vi "AMI_String_Field Z.vi"(8 "error in (no error)":errorcluster, 11 "String":string="Set Z Axis Magnetic Field 0.100Tesla at 0.030Tesla/min, PAUSE, Wait") -> (0 "error out":errorcluster, 2 "Z Rate":dbl, 3 "Z Field":dbl, 4 "Z H.Wait Stability":bool, 5 "Z Modo Rampa":u16(ring)=1 items=["RAMP", "PAUSE", "PAUSE", "MANUAL DOWN", "ZERO"])   [LabVIEW 2017]
panel:
  out "subString":string
  # "Set Z Axis Magnetic Field 0.100Tesla at 0.030Tesla/min, PAUSE, Wait"
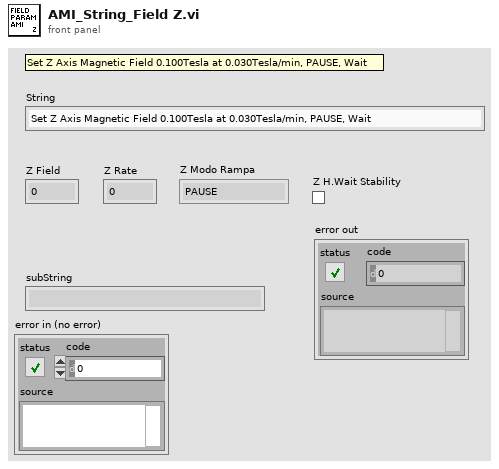
[diagram p1: front panel]
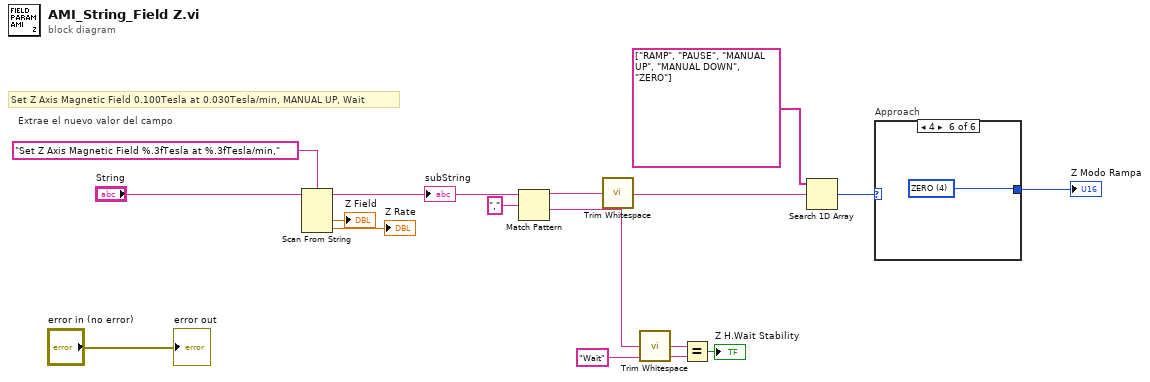
[diagram p0: block diagram]
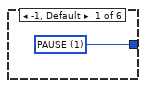
[diagram p2: hidden frame]
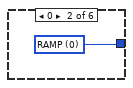
[diagram p3: hidden frame]
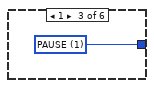
[diagram p4: hidden frame]
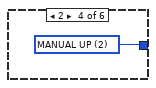
[diagram p5: hidden frame]
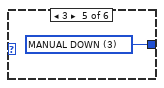
[diagram p6: hidden frame]
diagram:
  # "Set Z Axis Magnetic Field 0.100Tesla at 0.030Tesla/min, MANUAL UP, Wait"
  # "Extrae el nuevo valor del campo"
  n1 = Scan From String(format string="Set Z Axis Magnetic Field %.3fTesla at %.3fTesla/min,", input string="String") -> (remaining string=w5:string, output 1=→"Z Field":dbl, output 2=→"Z Rate":dbl)  [unwired: 4 in, 2 out]
  "subString" <- w5
  n2 = Match Pattern(string=w5, regular expression=",") -> (before substring=w7:string, after substring=w4:string)  [unwired: 1 in, 2 out]
  n3 = call <vilib>:"Trim Whitespace.vi"("string"=w7) -> ("trimmed string"=w2:string)  [unwired: 1 in]
  n4 = call <vilib>:"Trim Whitespace.vi"("string"=w4) -> ("trimmed string"=w6:string)  [unwired: 1 in]
  n5 = Equal?(x=w6, y="Wait" ("after substring")) -> (x = y?=→"Z H.Wait Stability":bool)
  n6 = Search 1D Array(1D array=string[] ["RAMP", "PAUSE", "MANUAL UP", "MANUAL DOWN", "ZERO"], element=w2) -> (index of element=w12:i32)  [unwired: 1 in]
  n7 = case "Approach" shown="4" w12 {
    tunnel: [w17 w18 w19 w20 w21 w22] -> w3
    frame -1, Default {
      w17 = u16 1 items=["RAMP", "PAUSE", "MANUAL UP", "MANUAL DOWN", "ZERO"] ("Modo Rampa")
    }
    frame 0 {
      w18 = u16 0 items=["RAMP", "PAUSE", "MANUAL UP", "MANUAL DOWN", "ZERO"] ("Modo Rampa")
    }
    frame 1 {
      w19 = u16 1 items=["RAMP", "PAUSE", "MANUAL UP", "MANUAL DOWN", "ZERO"] ("Modo Rampa")
    }
    frame 2 {
      w20 = u16 2 items=["RAMP", "PAUSE", "MANUAL UP", "MANUAL DOWN", "ZERO"] ("Modo Rampa")
    }
    frame 3 {
      w21 = u16 3 items=["RAMP", "PAUSE", "MANUAL UP", "MANUAL DOWN", "ZERO"] ("Modo Rampa")
    }
    frame 4 {
      w22 = u16 4 items=["RAMP", "PAUSE", "MANUAL UP", "MANUAL DOWN", "ZERO"] ("Modo Rampa")
    }
  }
  "Z Modo Rampa" <- w3
  "error out" <- "error in (no error)"
